vi "[FPGA] DeltaSig Main V6.vi"() -> ()   [LabVIEW 2015]
doc: "This VI provides a template for customizing a waveform acquisition using delta-sigma based NI C Series analog input smodules."
uses:
  <vilib>/eio/EIONode/EIONode.xnode
  <vilib>/eio/EIOPropertyNode/EIOPropertyNode.xnode
  <vilib>/rvi/DataTransferAndStorage/Container/XNode/niFpgaContainer.xnode
  <vilib>/rvi/eio/common/nirviEmuTemplateMethod_errors.vi
  <vilib>/rvi/eio/common/nirviEmuTemplatePropertyGet_errors.vi
  <vilib>/rvi/eio/common/nirviEmuTemplatePropertyGet_noerrors.vi
  <vilib>/rvi/eio/common/nirviEmuTemplatePropertySet_errors.vi
  <vilib>/rvi/eio/common/nirviEmuTemplatePropertySet_noerrors.vi
  <vilib>/LabVIEW Targets/FPGA/cRIO/shared/nicrio_ModuleControls/nicrio_cRIO-9234_ConfigModeRing.ctl
  <vilib>/LabVIEW Targets/FPGA/cRIO/shared/nicrio_ModuleControls/nicrio_cRIO-9234_DataRatesRing2.ctl
  <vilib>/LabVIEW Targets/FPGA/cRIO/shared/nicrio_DsaDataRateApi/_nicrio_9234GetDataRate131.vi
  <vilib>/rvi/interface/RandomDataEmulation/nirviRandomDataFpgaReadWriteTemplate.vi
panel:
  in  "Array Input Config":T1[](array[typedef])=[0, 0, 0, 0, 0, 0, 0, 0, 0, 0, 0, 0, 0, 0, 0, 0, 0, 0, 0, 0, 0, 0, 0, 0] items=["AC Coupled", "DC Coupled", "IEPE AC Coupled"]
  out "oclk freq":u32
  out "oclk div":u32
  out "oclk mult":u32
  in  "data rate (S/s)":u32
  in  "Chan Scale Array":sgl[](array[numeric])=[0.0, 0.0, 0.0, 0.0, 0.0, 0.0, 0.0, 0.0, 0.0, 0.0, 0.0, 0.0, 0.0, 0.0, 0.0, 0.0, 0.0, 0.0, 0.0, 0.0, 0.0, 0.0, 0.0, 0.0, 0.0, 0.0, 0.0, 0.0, 0.0, 0.0, 0.0, 0.0, 0.0, 0.0, 0.0, 0.0, 0.0, 0.0, 0.0, 0.0]
  out "Chan Count":bool
  out "Acq Loop Ticks":u32
  out "FPGA Error":errorcluster
  out "Module Underflow":bool
  out "Finished":bool
  in  "Number of Channels":i32=24
  in  "Samps per Chan [Finite]":i32=5120
  out "First Read":bool
  in  "Acquisition Type":enum16{"Finite Samples", "Continuous Samples"}(ring)
  out "DMA FIFO Full":bool
  in  "stop":bool
  # "Array size fixed at 40\nelements but may be \nexpanded if needed"
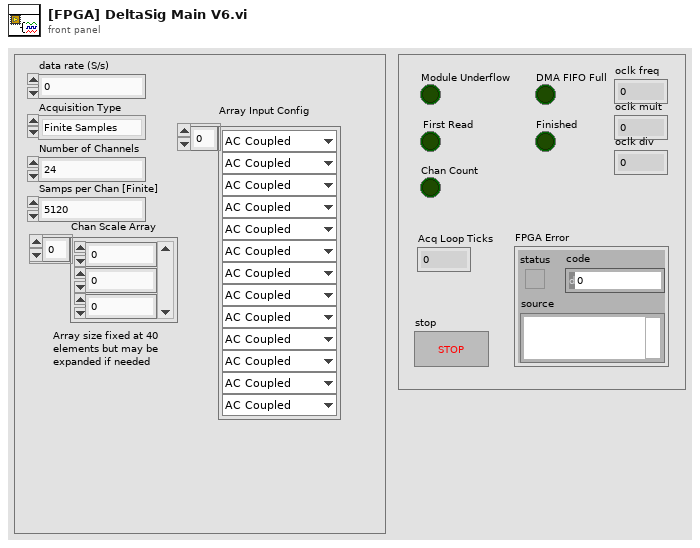
[diagram p1: front panel]
types:
  T1 = typedef "nicrio_cRIO-9234_ConfigModeRing.ctl" = u8
  T2 = typedef "nicrio_cRIO-9234_DataRatesRing2.ctl" = u8
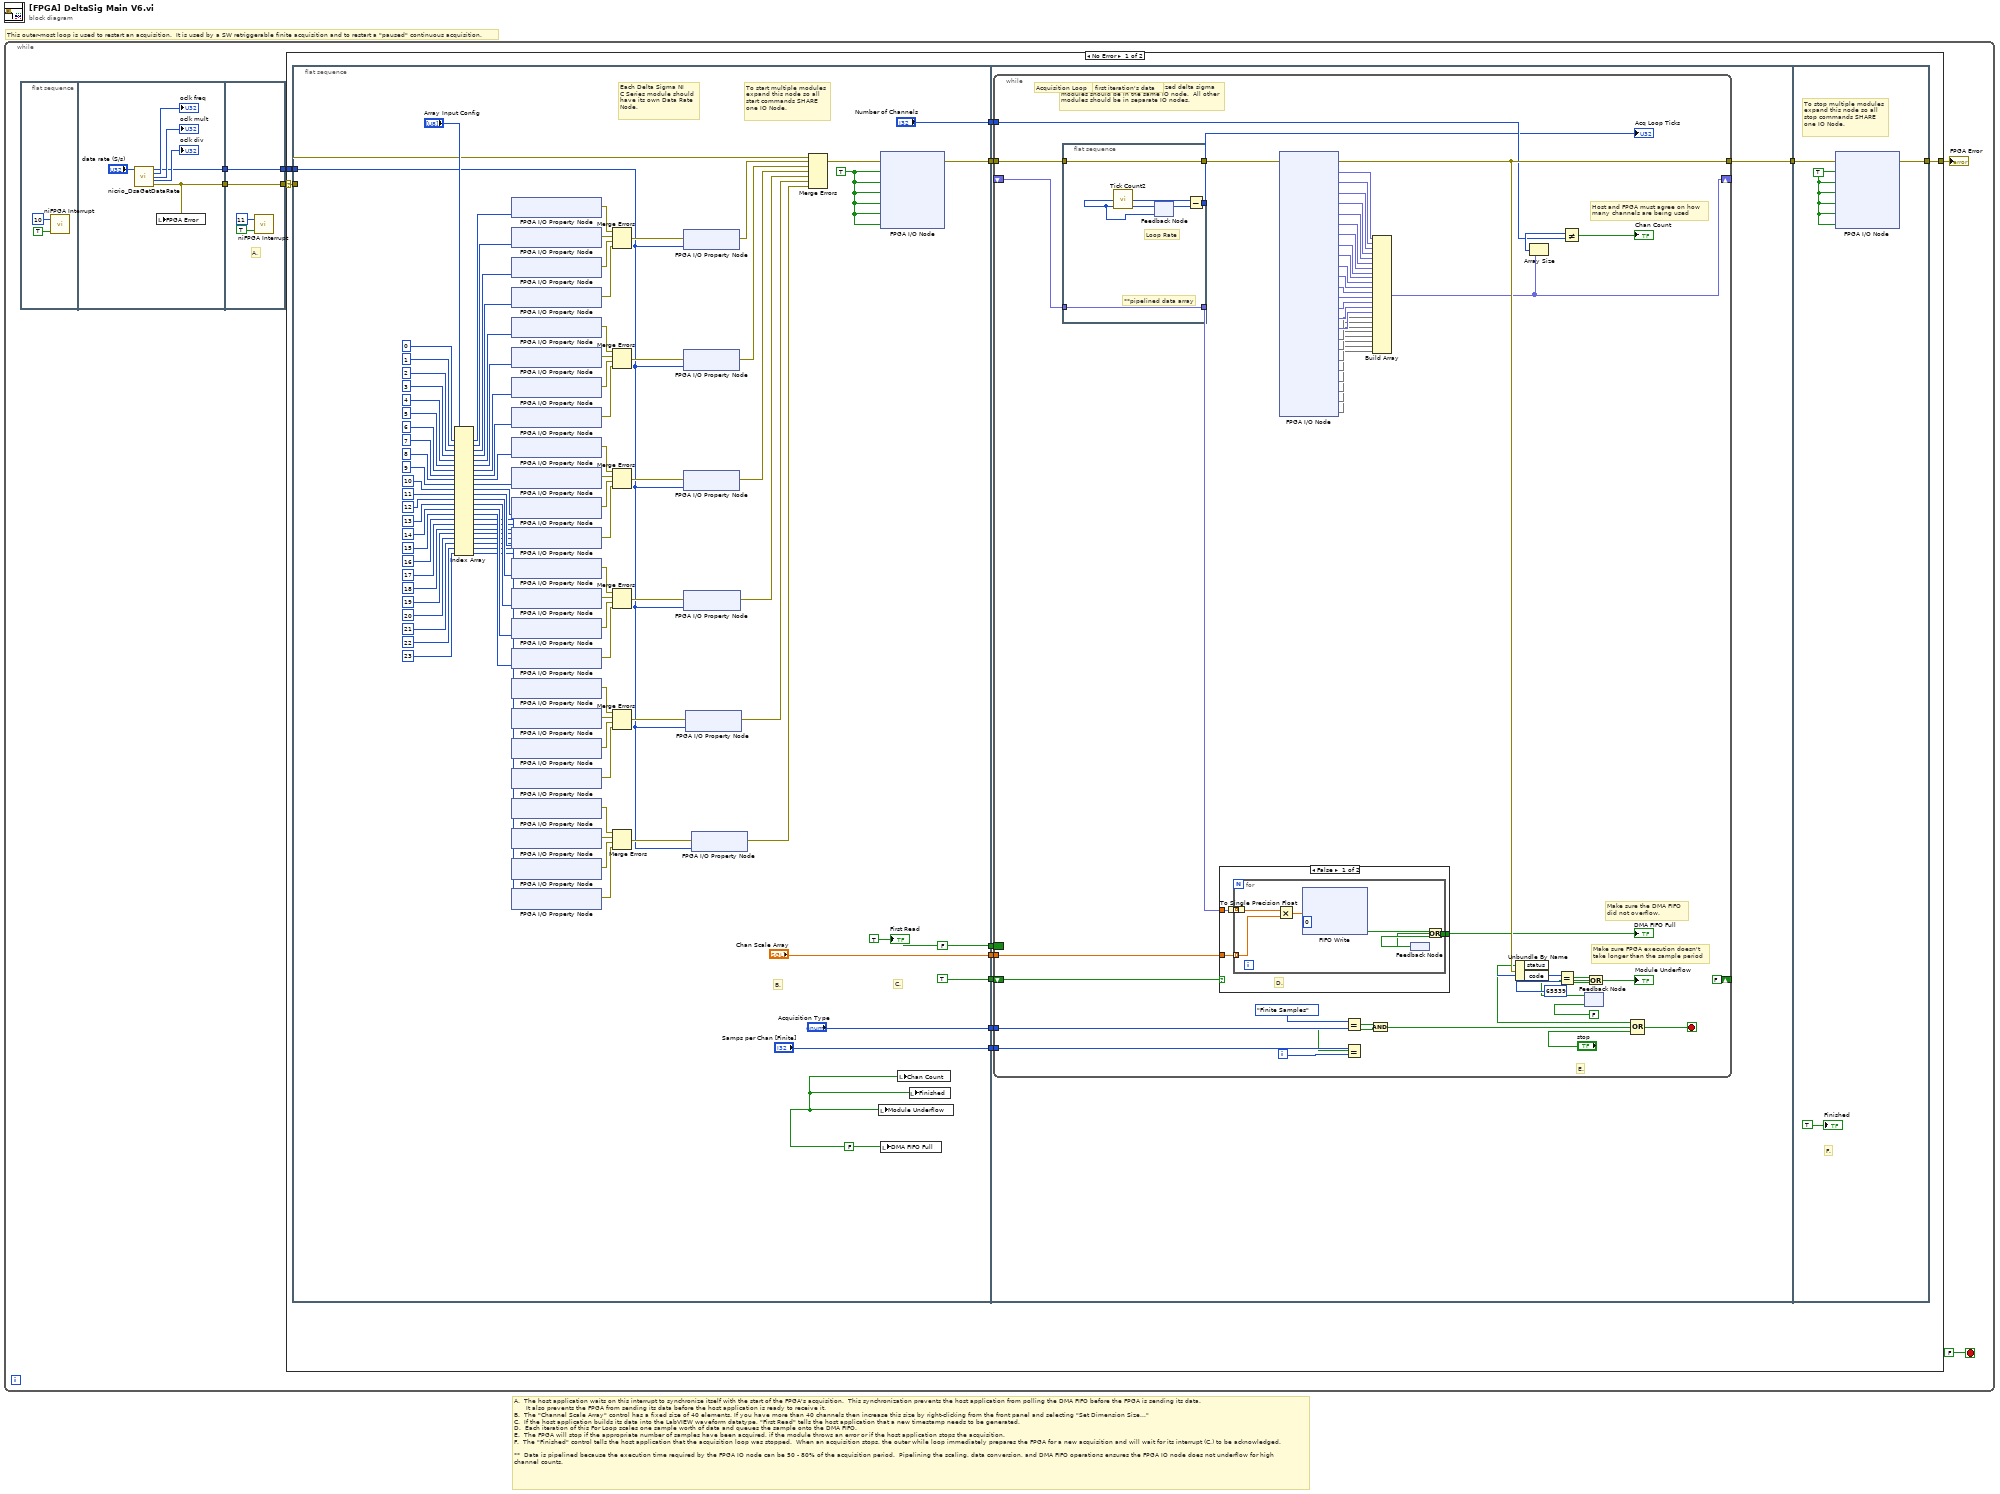
[diagram p0: block diagram]
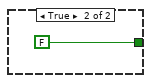
[diagram p2: hidden frame]
diagram:
  # "A.  The host application waits on this interrupt to synchronize itself with the start of the FPGA's acquisition.  This synchronization prevents the host application from polling the DMA FIFO before the FPGA is sending its data.\n      It also prevents the FPGA from sending its data before the host application is ready to receive it.\nB.  The \"Channel Scale Array\" control has a fixed size of 40 elements. If you have more than 40 channels then increase this size by right-clicking from the front panel and selecting \"Set Dimension Size...\"\nC.  If the host application builds its data into the LabVIEW waveform datatype, \"First Read\" tells the host application that a new timestamp needs to be generated.\nD.  Each iteration of this For Loop scales one sample worth of data and queues the sample onto the DMA FIFO.  \nE.  The FPGA will stop if the appropriate number of samples have been acquired, if the module throws an error or if the host application stops the acquisition.  \nF.  The \"Finished\" control tells the host application that the acquisition loop was stopped.  When an acquisition stops, the outer while loop immediately prepares the FPGA for a new acquisition and will wait for its interrupt (C.) to be acknowledged.\n\n**  Data is pipelined because the execution time required by the FPGA IO node can be 50 - 80% of the acquisition period.  Pipelining the scaling, data conversion, and DMA FIFO operations ensures the FPGA IO node does not underflow for high\nchannel counts."
  # "This outer-most loop is used to restart an acquisition.  It is used by a SW retriggerable finite acquisition and to restart a \"paused\" continuous acquisition."
  n1 = while {
    stop <- FALSE stop-if-true
    n2 = flat-sequence {
      tunnel: [w10] -> w2
      tunnel: [w11] -> w1
      tunnel: [w18] -> w3
      tunnel: [w15] -> w4
      tunnel: w2 -> [w15]
      tunnel: w1 -> [w18]
      frame #0 {
        n3 = call <vilib>:"niFPGA Interrupt.vi"("Wait Until Cleared (F)"=TRUE ("Wait Until Cleared"), "IRQ Number (0)"=u8 10 ("IRQ Number")) -> ()  [unwired: 1 in]
      }
      frame #1 {
        n4 = call-poly <vilib>:"nicrio_DsaGetDataRate.vi"("data rate (S/s)"="data rate (S/s)") -> ("data rate"=w11:T2, "oclk freq"=→"oclk freq":u32, "oclk mult"=→"oclk mult":u32, "oclk div"=→"oclk div":u32, "error out"=w10:errorcluster)  [unwired: 10 in]
        n5 = local write "FPGA Error"(w10) -> ()
      }
      frame #2 {
        # "A."
        n6 = call <vilib>:"niFPGA Interrupt.vi"("Wait Until Cleared (F)"=TRUE ("Wait Until Cleared"), "IRQ Number (0)"=u8 11 ("IRQ Number")) -> ()  [unwired: 1 in]
      }
    }
    n7 = case shown="No Error" w4 {
      selector: w4 -> [w19 w211]
      tunnel: [w21 w211] -> w5
      tunnel: w3 -> [w20 _]
      frame No Error {
        n8 = flat-sequence {
          tunnel: [w127] -> w29
          tunnel: ["Chan Scale Array"] -> w28
          tunnel: ["Acquisition Type"] -> w27
          tunnel: ["Samps per Chan [Finite]"] -> w26
          tunnel: ["Number of Channels"] -> w25
          tunnel: [TRUE ("t")] -> w24
          tunnel: [FALSE] -> w23
          tunnel: w20 -> [w34]
          tunnel: w19 -> [w99]
          tunnel: w29 -> [w134]
          tunnel: w28 -> [w133]
          tunnel: w27 -> [w131]
          tunnel: w26 -> [w130]
          tunnel: w25 -> [w135]
          tunnel: w24 -> [w132]
          tunnel: [w129] -> w22
          tunnel: w23 -> [w128]
          tunnel: w22 -> [w209]
          tunnel: [w208] -> w21
          frame #0 {
            w125 = FALSE ("Module Underflow")
            w87 = TRUE ("Mod1/Start")
            # "To start multiple modules\nexpand this node so all\nstart commands SHARE\none IO Node."
            # "C."
            # "B."
            # "Each Delta Sigma NI \nC Series module should \nhave its own Data Rate \nNode."
            n9 = Index Array(array="Array Input Config", index #1=0 ("index"), index #2=1 ("index"), index #3=2 ("index"), index #4=3 ("index"), index #5=4 ("index"), index #6=5 ("index"), index #7=6 ("index"), index #8=7 ("index"), index #9=8 ("index"), index #10=9 ("index"), index #11=10 ("index"), index #12=11 ("index"), index #13=12 ("index"), index #14=13 ("index"), index #15=14 ("index"), index #16=15 ("index"), index #17=16 ("index"), index #18=17 ("index"), index #19=18 ("index"), index #20=19 ("index"), index #21=20 ("index"), index #22=21 ("index"), index #23=22 ("index"), index #24=23 ("index")) -> (element #1=w117:T1, element #2=w116:T1, element #3=w115:T1, element #4=w114:T1, element #5=w95:T1, element #6=w94:T1, element #7=w93:T1, element #8=w92:T1, element #9=w74:T1, element #10=w73:T1, element #11=w72:T1, element #12=w71:T1, element #13=w70:T1, element #14=w68:T1, element #15=w67:T1, element #16=w66:T1, element #17=w65:T1, element #18=w64:T1, element #19=w63:T1, element #20=w62:T1, element #21=w45:T1, element #22=w44:T1, element #23=w43:T1, element #24=w42:T1)
            n10 = xnode "FPGA I/O Property Node"("Input Configuration"=w117) -> ("error out"=w110:errorcluster)  [unwired: 2 in, 1 out]
            n11 = xnode "FPGA I/O Property Node"("Input Configuration"=w116) -> ("error out"=w109:errorcluster)  [unwired: 2 in, 1 out]
            n12 = xnode "FPGA I/O Property Node"("Input Configuration"=w115) -> ("error out"=w108:errorcluster)  [unwired: 2 in, 1 out]
            n13 = xnode "FPGA I/O Property Node"("Input Configuration"=w114) -> ("error out"=w107:errorcluster)  [unwired: 2 in, 1 out]
            n14 = xnode "FPGA I/O Property Node"("Input Configuration"=w95) -> ("error out"=w104:errorcluster)  [unwired: 2 in, 1 out]
            n15 = xnode "FPGA I/O Property Node"("Input Configuration"=w94) -> ("error out"=w103:errorcluster)  [unwired: 2 in, 1 out]
            n16 = xnode "FPGA I/O Property Node"("Input Configuration"=w93) -> ("error out"=w102:errorcluster)  [unwired: 2 in, 1 out]
            n17 = xnode "FPGA I/O Property Node"("Input Configuration"=w92) -> ("error out"=w101:errorcluster)  [unwired: 2 in, 1 out]
            n18 = xnode "FPGA I/O Property Node"("Input Configuration"=w74) -> ("error out"=w86:errorcluster)  [unwired: 2 in, 1 out]
            n19 = xnode "FPGA I/O Property Node"("Input Configuration"=w73) -> ("error out"=w85:errorcluster)  [unwired: 2 in, 1 out]
            n20 = xnode "FPGA I/O Property Node"("Input Configuration"=w72) -> ("error out"=w84:errorcluster)  [unwired: 2 in, 1 out]
            n21 = xnode "FPGA I/O Property Node"("Input Configuration"=w71) -> ("error out"=w83:errorcluster)  [unwired: 2 in, 1 out]
            n22 = xnode "FPGA I/O Property Node"("Input Configuration"=w70) -> ("error out"=w82:errorcluster)  [unwired: 2 in, 1 out]
            n23 = xnode "FPGA I/O Property Node"("Input Configuration"=w68) -> ("error out"=w81:errorcluster)  [unwired: 2 in, 1 out]
            n24 = xnode "FPGA I/O Property Node"("Input Configuration"=w67) -> ("error out"=w80:errorcluster)  [unwired: 2 in, 1 out]
            n25 = xnode "FPGA I/O Property Node"("Input Configuration"=w66) -> ("error out"=w79:errorcluster)  [unwired: 2 in, 1 out]
            n26 = xnode "FPGA I/O Property Node"("Input Configuration"=w65) -> ("error out"=w78:errorcluster)  [unwired: 2 in, 1 out]
            n27 = xnode "FPGA I/O Property Node"("Input Configuration"=w64) -> ("error out"=w77:errorcluster)  [unwired: 2 in, 1 out]
            n28 = xnode "FPGA I/O Property Node"("Input Configuration"=w63) -> ("error out"=w76:errorcluster)  [unwired: 2 in, 1 out]
            n29 = xnode "FPGA I/O Property Node"("Input Configuration"=w62) -> ("error out"=w75:errorcluster)  [unwired: 2 in, 1 out]
            n30 = xnode "FPGA I/O Property Node"("Input Configuration"=w45) -> ("error out"=w49:errorcluster)  [unwired: 2 in, 1 out]
            n31 = xnode "FPGA I/O Property Node"("Input Configuration"=w44) -> ("error out"=w48:errorcluster)  [unwired: 2 in, 1 out]
            n32 = xnode "FPGA I/O Property Node"("Input Configuration"=w43) -> ("error out"=w47:errorcluster)  [unwired: 2 in, 1 out]
            n33 = xnode "FPGA I/O Property Node"("Input Configuration"=w42) -> ("error out"=w46:errorcluster)  [unwired: 2 in, 1 out]
            n34 = Merge Errors(w110, w109, w108, w107) -> (w106:errorcluster)
            n35 = Merge Errors(w104, w103, w102, w101) -> (w100:errorcluster)
            n36 = Merge Errors(w86, w85, w84, w83) -> (w69:errorcluster)
            n37 = Merge Errors(w82, w81, w80, w79) -> (w37:errorcluster)
            n38 = Merge Errors(w78, w77, w76, w75) -> (w36:errorcluster)
            n39 = Merge Errors(w49, w48, w47, w46) -> (w35:errorcluster)
            n40 = xnode "FPGA I/O Property Node"("error in"=w106, "Data Rate"=w34) -> ("error out"=w97:errorcluster)  [unwired: 1 in, 1 out]
            n41 = xnode "FPGA I/O Property Node"("error in"=w100, "Data Rate"=w34) -> ("error out"=w96:errorcluster)  [unwired: 1 in, 1 out]
            n42 = xnode "FPGA I/O Property Node"("error in"=w69, "Data Rate"=w34) -> ("error out"=w33:errorcluster)  [unwired: 1 in, 1 out]
            n43 = xnode "FPGA I/O Property Node"("error in"=w37, "Data Rate"=w34) -> ("error out"=w32:errorcluster)  [unwired: 1 in, 1 out]
            n44 = xnode "FPGA I/O Property Node"("error in"=w36, "Data Rate"=w34) -> ("error out"=w31:errorcluster)  [unwired: 1 in, 1 out]
            n45 = xnode "FPGA I/O Property Node"("error in"=w35, "Data Rate"=w34) -> ("error out"=w30:errorcluster)  [unwired: 1 in, 1 out]
            n46 = Merge Errors(w99, w97, w96, w33, w32, w31, w30) -> (w98:errorcluster)
            n47 = local write "Module Underflow"(w125) -> ()
            n48 = xnode "FPGA I/O Node"("error in"=w98, "Mod1/Start"=w87, "Mod2/Start"=w87, "Mod3/Start"=w87, "Mod4/Start"=w87, "Mod5/Start"=w87, "Mod6/Start"=w87) -> ("error out"=w127:errorcluster)  [unwired: 6 in, 6 out]
            n49 = local write "DMA FIFO Full"(w125) -> ()
            n50 = local write "Chan Count"(w125) -> ()
            n51 = local write "Finished"(w125) -> ()
            "First Read" <- TRUE ("First Read")
          }
          frame #1 {
            n52 = while {
              tunnel: w134 -> [w179]
              tunnel: [w184] -> w129
              tunnel: w131 -> [w186]
              tunnel: w130 -> [w185]
              shift-right: [w159] -> _
              shift-left: _ -> [w172]
              tunnel: w135 -> [w181]
              tunnel: w133 -> [w173]
              shift-right: [FALSE ("t")] -> _
              shift-left: w132 -> [w171]
              border: w128 -> [_]
              i -> [w169]
              stop <- w156 stop-if-true
              # "Add channels here.  All synchronized delta sigma\nmodules should be in the same IO node.  All other\nmodules should be in separate IO nodes."
              # "Do not DMA first iteration's data"
              # "Acquisition Loop"
              # "E."
              # "Host and FPGA must agree on how \nmany channels are being used"
              # "Make sure the DMA FIFO\ndid not overflow."
              # "Make sure FPGA execution doesn't\ntake longer than the sample period"
              n53 = flat-sequence {
                tunnel: [w206] -> w178
                tunnel: w179 -> [w206]
                tunnel: [w203] -> w177
                tunnel: w172 -> [w202]
                tunnel: [w202] -> w158
                frame #0 {
                  # "**pipelined data array"
                  # "Loop Rate"
                  n54 = call "Tick Count2"() -> ("Tick Count(Ticks)"=w205:u32)
                  n55 = feedback-in #1(w205) -> ()
                  n56 = feedback #1(w205) -> (w204:u32)
                  n57 = Subtract(x=w205, y=w204) -> (x-y=w203:u32)
                }
              }
              n58 = To Single Precision Float(number=w158) -> (single precision float=w157:sgl[])
              n59 = case shown="False" w171 {
                tunnel: [w193 FALSE] -> w183
                tunnel: w173 -> [w192 _]
                tunnel: w157 -> [w191 _]
                frame False {
                  # "D."
                  n60 = for {
                    tunnel: [w198] -> w193
                    tunnel: w191 -> [w196] mode=indexing
                    tunnel: w192 -> [w195] mode=indexing
                    n61 = Multiply(x=w196, y=w195) -> (x*y=w194:sgl)
                    n62 = xnode ("FIFO Write")("Element"=w194, "Timeout"=0) -> ("Timed Out?"=w200:bool)  [unwired: 1 in, 1 out]
                    n63 = feedback #2() -> (w199:bool)
                    n64 = Or(x=w200, y=w199) -> (x .or. y?=w198:bool)
                    n65 = feedback-in #2(w198) -> ()
                  }
                }
                frame True {
                }
              }
              "DMA FIFO Full" <- w183
              n66 = xnode "FPGA I/O Node"("error in"=w178) -> ("error out"=w184:errorcluster, "Mod1/AI0"=w176:fxp<+/-,24,4>, "Mod1/AI1"=w168:fxp<+/-,24,4>, "Mod1/AI2"=w175:fxp<+/-,24,4>, "Mod1/AI3"=w174:fxp<+/-,24,4>, "Mod2/AI0"=w155:fxp<+/-,24,4>, "Mod2/AI1"=w154:fxp<+/-,24,4>, "Mod2/AI2"=w153:fxp<+/-,24,4>, "Mod2/AI3"=w152:fxp<+/-,24,4>, "Mod3/AI0"=w151:fxp<+/-,24,4>, "Mod3/AI1"=w150:fxp<+/-,24,4>, "Mod3/AI2"=w149:fxp<+/-,24,4>, "Mod3/AI3"=w148:fxp<+/-,24,4>, "Mod4/AI0"=w147:fxp<+/-,24,4>, "Mod4/AI1"=w146:fxp<+/-,24,4>, "Mod4/AI2"=w145:fxp<+/-,24,4>, "Mod4/AI3"=w144:fxp<+/-,24,4>, "Mod5/AI0"=w143, "Mod5/AI1"=w142, "Mod5/AI2"=w141, "Mod5/AI3"=w140, "Mod6/AI0"=w139, "Mod6/AI1"=w138, "Mod6/AI2"=w137, "Mod6/AI3"=w136)  [unwired: 24 in, 24 out]
              n67 = Equal?(x=enum16{"Finite Samples", "Continuous Samples"}."Finite Samples" ("y"), y=w186) -> (x = y?=w162:bool)
              n68 = Equal?(x=w185, y=w169) -> (x = y?=w161:bool)
              n69 = And(x=w162, y=w161) -> (x .and. y?=w160:bool)
              n70 = Build Array(w176, w168, w175, w174, w155, w154, w153, w152, w151, w150, w149, w148, w147, w146, w145, w144, w143, w142, w141, w140, w139, w138, w137, w136) -> (w159:fxp<+/-,24,4>[])
              n71 = Unbundle By Name(w184) -> ("status"=w167:bool, "code"=w187:i32)
              n72 = Array Size(array=w159) -> (size(s)=w182:i32)
              n73 = Equal?(x=w187, y=65539) -> (x = y?=w164:bool)
              n74 = Not Equal?(x=w182, y=w181) -> (x != y?=→"Chan Count":bool)
              n75 = feedback #3(FALSE) -> (w166:bool)
              n76 = Or(x=w164, y=w166) -> (x .or. y?=w163:bool)
              "Module Underflow" <- w163
              n77 = feedback-in #3(w163) -> ()
              n78 = Compound Arithmetic op=OR(w167, w160, "stop") -> (w156:bool)
              "Acq Loop Ticks" <- w177
            }
          }
          frame #2 {
            w207 = TRUE ("Mod1/Stop")
            # "To stop multiple modules\nexpand this node so all\nstop commands SHARE\none IO Node."
            # "F."
            n79 = xnode "FPGA I/O Node"("error in"=w209, "Mod1/Stop"=w207, "Mod2/Stop"=w207, "Mod3/Stop"=w207, "Mod4/Stop"=w207, "Mod5/Stop"=w207, "Mod6/Stop"=w207) -> ("error out"=w208:errorcluster)  [unwired: 6 in, 6 out]
            "Finished" <- TRUE ("Finished")
          }
        }
      }
      frame Error {
      }
    }
    "FPGA Error" <- w5
  }
